vi "Configure Ref Clock Source Core.vi"(8 "error in (no error)":errorcluster, 9 "reference clock source (Internal)":i32(ring) items=["Internal"=0, "External"=1, "RTSI Clock"=101], 11 "IVI_Fgen in":refnum<class "IVI_Fgen.lvclass">) -> (0 "error out":errorcluster, 3 "IVI_Fgen out":refnum<class "IVI_Fgen.lvclass">)   [LabVIEW 2013, in "IVI_Fgen.lvlib" / "IVI_Fgen.lvclass"]
doc: "This VI configures the function generator's reference clock source. The function generator uses the reference clock to derive frequencies and sample rates when generating output."
uses:
  IVI_Fgen.lvclass
  IVI_Fgen.lvclass/IVI_Fgen.ctl
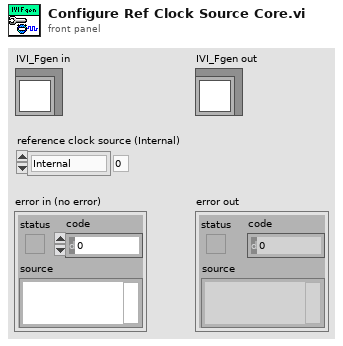
[diagram p1: front panel]
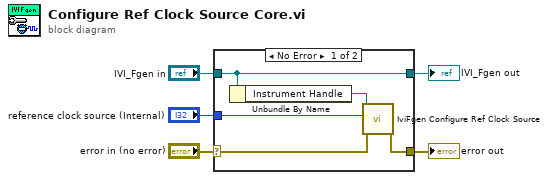
[diagram p0: block diagram]
diagram:
  n1 = case shown="No Error" "error in (no error)" {
    selector: "error in (no error)" -> [w8 w12]
    tunnel: [w7 w12] -> w4
    tunnel: [w10 w11] -> w2
    tunnel: "IVI_Fgen in" -> [w10 w11]
    tunnel: "reference clock source (Internal)" -> [w6 _]
    frame No Error {
      n2 = Unbundle By Name(w10) -> ("Instrument Handle"=w9:refnum<k15>)
      n3 = call <vilib>:"IviFgen Configure Ref Clock Source.vi"("error in (no error)"=w8, "reference clock source (Internal)"=w6, "instrument handle"=w9) -> ("error out"=w7:errorcluster)  [unwired: 7 in, 1 out]
    }
    frame Error {
    }
  }
  "error out" <- w4
  "IVI_Fgen out" <- w2
